vi "lab session 6.1.vi"() -> ()   [LabVIEW 2020]
uses:
  <vilib>/numeric/Random Number (Range) U64.vi
  <vilib>/numeric/sub_Random U32.vi
panel:
  out "Array 2":dbl[][](array[numeric])
  in  "Array":dbl[](array[numeric])
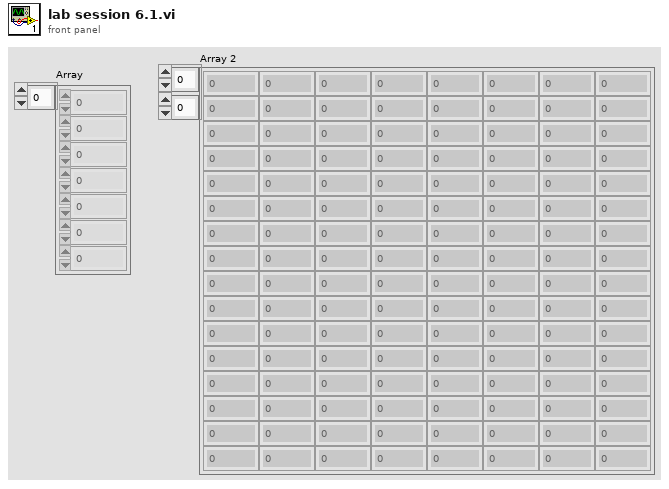
[diagram p1: front panel]
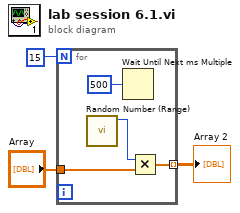
[diagram p0: block diagram]
diagram:
  n1 = for {
    N: 15 -> [_]
    tunnel: "Array" -> [w7]
    tunnel: [w5] -> w1 mode=indexing
    n2 = call-poly <vilib>:"Random Number (Range).vi"() -> ("number"=w4:u64)  [unwired: 11 in]
    n3 = Wait Until Next ms Multiple(millisecond multiple=u32 500) -> ()  [unwired: 1 out]
    n4 = Multiply(x=w4, y=w7) -> (x*y=w5:dbl[])
  }
  "Array 2" <- w1
